vi "Add pipe.vi"(0 "Add?":bool) -> ()   [LabVIEW 2014]
uses:
  Labby Bird/Labby Bird/Labby bird-Support.llb/Global-1.vi
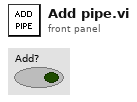
[diagram p1: front panel]
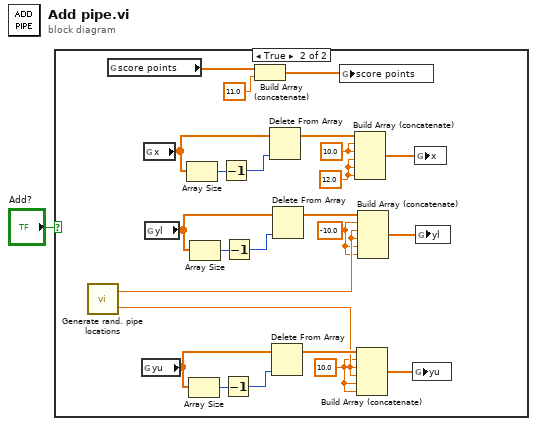
[diagram p0: block diagram]
diagram:
  n1 = case shown="True" "Add?" {
    frame False {
    }
    frame True {
      w2 = 10.0
      w3 = -10.0
      w4 = 12.0
      w21 = 10.0
      n2 = call "Generate rand. pipe locations.vi"() -> ("lower"=w14:dbl, "upper"=w8:dbl)  [unwired: 1 in]
      n3 = global read "Global-1.vi" "score points"() -> (w7:dbl[])
      n4 = global read "Global-1.vi" "yu"() -> (w13:dbl[])
      n5 = global read "Global-1.vi" "x"() -> (w25:dbl[])
      n6 = global read "Global-1.vi" "yl"() -> (w19:dbl[])
      n7 = Array Size(array=w25) -> (size(s)=w24:i32)
      n8 = Array Size(array=w13) -> (size(s)=w12:i32)
      n9 = Array Size(array=w19) -> (size(s)=w18:i32)
      n10 = Decrement(x=w24) -> (x-1=w23:i32)
      n11 = Decrement(x=w12) -> (x-1=w11:i32)
      n12 = Decrement(x=w18) -> (x-1=w17:i32)
      n13 = Build Array (concatenate)(w7, 11.0) -> (w6:dbl[])
      n14 = Delete From Array(array=w25, index=w23) -> (array with subset deleted=w22:dbl[])  [unwired: 1 in, 1 out]
      n15 = Delete From Array(array=w13, index=w11) -> (array with subset deleted=w10:dbl[])  [unwired: 1 in, 1 out]
      n16 = Delete From Array(array=w19, index=w17) -> (array with subset deleted=w16:dbl[])  [unwired: 1 in, 1 out]
      n17 = global write "Global-1.vi" "score points"(w6) -> ()
      n18 = Build Array (concatenate)(w22, w21, w21, w4, w4, w4) -> (w20:dbl[])
      n19 = Build Array (concatenate)(w10, w2, w8, w8, w2, w2) -> (w9:dbl[])
      n20 = Build Array (concatenate)(w16, w3, w14, w14, w3, w3) -> (w15:dbl[])
      n21 = global write "Global-1.vi" "yu"(w9) -> ()
      n22 = global write "Global-1.vi" "x"(w20) -> ()
      n23 = global write "Global-1.vi" "yl"(w15) -> ()
    }
  }
